vi "Control Path.vi"(11 "BooleanIndicatorEditorPanel in":refnum<class "BooleanIndicatorEditorPanel.lvclass">) -> (2 "Control Paths":path[](array[path]))   [LabVIEW 2020, in "VolatusGUIControls.lvlib" / "BooleanIndicatorEditorPanel.lvclass"]
uses:
  BooleanIndicatorEditorPanel.lvclass
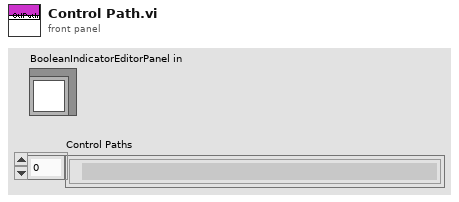
[diagram p1: front panel]
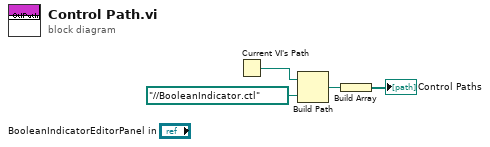
[diagram p0: block diagram]
diagram:
  n1 = Current VI's Path() -> (path=w4:path)
  n2 = Build Path(base path=w4, name or relative path=path "../../BooleanIndicator.ctl") -> (appended path=w2:path)
  n3 = Build Array(w2) -> (→"Control Paths":path[])
